vi "Person.vi"(0 "Person in":refnum<class "Person.lvclass">, 5 "name":string, 7 "gender":string, 9 "maritalStatus":string, 11 "error in (no error)":errorcluster) -> (4 "Person out":refnum<class "Person.lvclass">, 15 "error out":errorcluster)   [LabVIEW 2018, in "Person.lvclass"]
uses:
  Person.lvclass
  Person.lvclass/Person.ctl
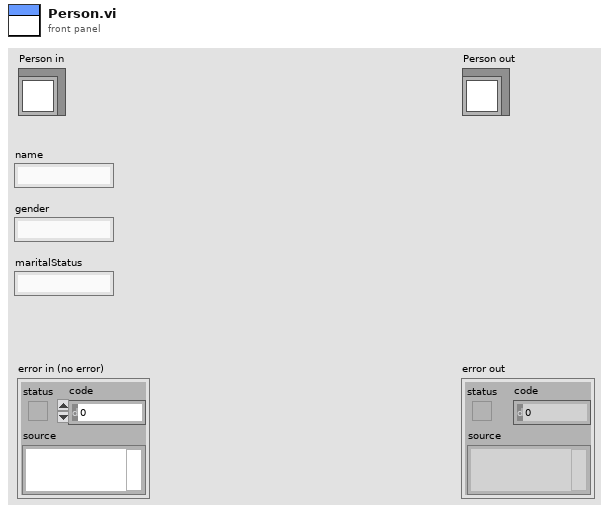
[diagram p1: front panel]
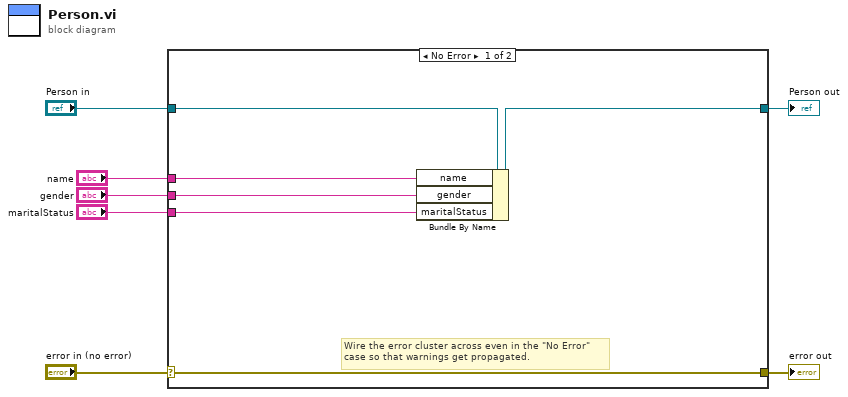
[diagram p0: block diagram]
diagram:
  n1 = case shown="No Error" "error in (no error)" {
    selector: "error in (no error)" -> [w12 w15]
    tunnel: [w12 w15] -> w6
    tunnel: [w11 w14] -> w4
    tunnel: "Person in" -> [w13 w14]
    tunnel: "maritalStatus" -> [w10 _]
    tunnel: "gender" -> [w9 _]
    tunnel: "name" -> [w8 _]
    frame No Error {
      # "Wire the error cluster across even in the \"No Error\"\ncase so that warnings get propagated."
      n2 = Bundle By Name(cluster=w13, "name"=w8, "gender"=w9, "maritalStatus"=w10) -> (w11:refnum<class "Person.lvclass">)
    }
    frame Error {
    }
  }
  "error out" <- w6
  "Person out" <- w4
